vi "Inverse2x2.vi"() -> ()   [LabVIEW 2015]
panel:
  in  "stop":bool
  out "Inverse Matrix":dbl[][](array[numeric])
  in  "2x2Matrix":dbl[][](array[numeric])
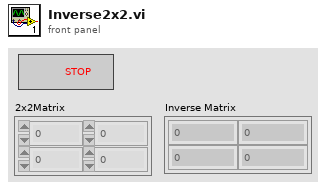
[diagram p1: front panel]
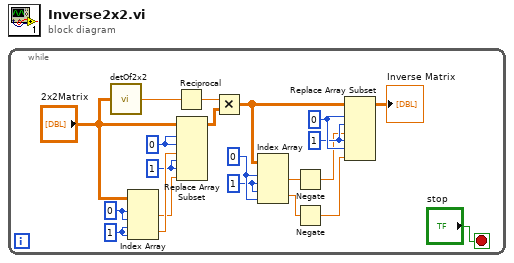
[diagram p0: block diagram]
diagram:
  n1 = while {
    stop <- "stop" stop-if-true
    w7 = 1 ("index (row)")
    w10 = 0 ("index (row)")
    w12 = 1 ("index (row)")
    w13 = 0 ("index (row)")
    w16 = 1 ("disabled index (col)")
    w17 = 0 ("index (row)")
    w18 = 1 ("disabled index (col)")
    w19 = 0 ("index (row)")
    n2 = call "detOf2x2.vi"("2x2Matrix"="2x2Matrix") -> ("Determinant"=w21:dbl)
    n3 = Index Array(array="2x2Matrix", index (row) #1=w13, index (col) #1=w13, index (row) #2=w12, index (col) #2=w12) -> (element #1=w8:dbl, element #2=w9:dbl)
    n4 = Reciprocal(x=w21) -> (1/x=w20:dbl)
    n5 = Replace Array Subset(array="2x2Matrix", new element #1=w9, index (row) #1=w10, index (col) #1=w10, new element #2=w8, index (row) #2=w7, index (col) #2=w7) -> (w6:dbl[][])
    n6 = Multiply(x=w20, y=w6) -> (x*y=w4:dbl[][])
    n7 = Index Array(array=w4, index (row) #1=w19, index (col) #1=w18, index (row) #2=w18, index (col) #2=w19) -> (element #1=w3:dbl, element #2=w2:dbl)
    n8 = Negate(x=w3) -> (-x=w15:dbl)
    n9 = Negate(x=w2) -> (-x=w14:dbl)
    n10 = Replace Array Subset(array=w4, new element #1=w15, index (row) #1=w17, index (col) #1=w16, new element #2=w14, index (row) #2=w16, index (col) #2=w17) -> (→"Inverse Matrix":dbl[][])
  }
